vi "PH_ImageOperator.FF MaxEnergy.vi"(0 "i ref in":refnum<vi>, 1 "Image":T1, 2 "Fill Factor":dbl, 5 "error in (no error)":errorcluster) -> (14 "i ref out":refnum<vi>, 16 "Max. allowed energy (J)":dbl, 17 "Error calculating the Energy?":bool, 19 "error out":errorcluster)   [LabVIEW 2014, in "PH_ImageOperator.lvlib"]
doc: "This VI calculates the maximum allowed energy based on a beam profile, the fill factor and a maximum damage threshold fluence.\nThe image to be fed in must be the binary image generated by the \"Convex Hull\" VI."
uses:
  PH_ImageOperator.lvlib
  <vilib>/vision/Image Controls.llb/IMAQ Image.ctl
  <vilib>/vision/NI_Vision_Development_Module.lvlib
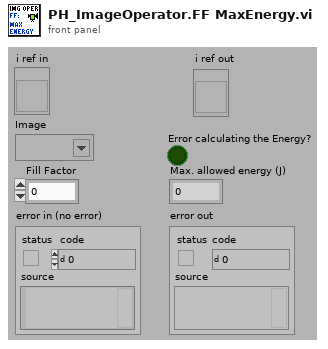
[diagram p1: front panel]
types:
  T1 = typedef "IMAQ Image.ctl" = refnum<image>
  T2 = typedef "PH_ImageOperator.lvlib/PH_ImageOperator.i attribute.ctl" = cluster{"GUI Refs":cluster{"Delete":refnum<vi>, "Calibration status":refnum<vi>, "BI subtracted":refnum<vi>, "calc Energy":refnum<vi>, "Energy: expected value":refnum<vi>, "Energy: Tolerance":refnum<vi>, "Energy calculated":refnum<vi>, "Energy":refnum<vi>, "calc Beam Anal":refnum<vi>, "Maj Diam 1/esquare":refnum<vi>, "Min Diam 1/esquare":refnum<vi>, "Azi Angle":refnum<vi>, "Min/Maj Diam esquare":refnum<vi>, "Beam analysed":refnum<vi>, "CoG - x":refnum<vi>, "CoG - y":refnum<vi>, "BA: Method":refnum<vi>, "BA: Steps":refnum<vi>, "BA: Factor":refnum<vi>, "calc Traces":refnum<vi>, "Traces: Fit Gauss":refnum<vi>, "Traces calculated":refnum<vi>, "Maj FWHM":refnum<vi>, "Min FWHM":refnum<vi>, "Major Trace":refnum<vi>, "Minor Trace":refnum<vi>, "Maj Fit Order":refnum<vi>, "Min Fit Order":refnum<vi>, "Position calculated":refnum<vi>, "Position":refnum<vi>, "Type":refnum<vi>, "Center":refnum<vi>, "exp - X":refnum<vi>, "exp - Y":refnum<vi>, "Tolerance":refnum<vi>, "f":refnum<vi>, "M":refnum<vi>, "D":refnum<vi>, "q":refnum<vi>, "Dummy Method":refnum<vi>, "Dummy Type":refnum<vi>, "Global On":refnum<vi>, "Traces: No offset":refnum<vi>, "Maj 99%":refnum<vi>, "Min 99%":refnum<vi>, "GUI FF Image":refnum<vi>, "calc Fill Factor":refnum<vi>, "FF calculated":refnum<vi>, "Fill Factor: Filter?":refnum<vi>, "FF: Damage Threshold":refnum<vi>, "FF: Threshold":refnum<vi>, "FF: max allow. Energy":refnum<vi>, "FF: Fillfactor":refnum<vi>, "Calibration data":refnum<vi>}, "List of GUIs":string[], "Calibration":cluster{"Status":T3, "Calibration data":T4, "Calibration Data File":path}, "Final Image":cluster{"BI Subtraction Failure":bool}, "Energy":cluster{"on":bool, "expected value [mJ]":dbl, "Tolerance [%]":dbl, "State":T3, "Energy [mJ]":dbl, "Unit":string, "calculated @":timestamp}, "Beam Analysis":cluster{"on":bool, "Data":T5, "Method":bool, "Steps":i32, "Factor":i32, "ROI":cluster{"Left":i32, "Top":i32, "Right":i32, "Bottom":i32}, "analysed @":timestamp}, "Trace Analysis":cluster{"on":bool, "Fit on":bool, "Maj FWHM":dbl, "Min FWHM":dbl, "Maj Fit Order":i32, "Min Fit Order":i32, "No Offset":bool, "Maj 99%":dbl, "Min 99%":dbl, "Traces":cluster{"XScaleName":string, "Y Scale Minimum":sgl, "Y Scale Maximum":sgl, "X Scale Minimum":sgl, "X Scale Maximum":sgl, "Traces":cluster{"Index":sgl[], "Trace":dbl[]}[]}[], "analysed @":timestamp}, "Position Analysis":cluster{"on":bool, "exp - X":i32, "exp - Y":i32, "focal length [mm]":dbl, "Magnification":dbl, "Delta":dbl, "Theta":dbl, "Tolerance":dbl, "Type":bool, "analysed @":timestamp}, "Fill Factor":cluster{"on":bool, "Filter on?":bool, "Threshold":dbl, "Damage Threshold [J/cm²]":dbl, "Fillfactor":dbl, "Max. allowed Energy [J]":dbl, "calculated @":timestamp}, "Statistician Service ID":i32, "Images":cluster{"Background":T1, "OP":T1, "GUI":T1, "BA: ROI":T1, "Trace: Turn":T1, "FF: Main":T1, "FF: Help":T1, "PSDB: BG":T1, "PSDB: OP":T1, "PSDB: FF":T1}}
  T3 = typedef "PH_StatusHandler.lvlib/PH_StatusHandler.Status.ctl" = i16
  T4 = typedef "PH_ImageCalibrator.lvlib/PH_ImageCalibrator.Calibration Data.ctl" = cluster{"Date":string, "Time":string, "Cam Settings":cluster{"Cam ID":string, "Gain":dbl, "Brightness":dbl, "Shutter":dbl, "Cam Error":bool, "Mode":i32}, "Background Image":cluster{"Image":dbl[][], "Image Error":bool}, "Linear Calibration":cluster{"Calibration Factor":dbl, "not mm or mrad":bool}, "Energy Calibration":cluster{"Calibration Factor":dbl, "no mJ":bool}}
  T5 = typedef "PH_ImageOperator.lvlib/PH_ImageOperator.Beam Analysis Data.ctl" = cluster{"CoG-x":sgl, "CoG-y":sgl, "Maj Dim":dbl, "Min Dim":dbl, "Ellipticity":dbl, "Azimuth Angle [rad]":dbl, "Azi Angle rel to Maj?":bool}
  T6 = cluster{"histogram":u32[], "Minimal Value":sgl, "Maximal Value":sgl, "Starting Value":sgl, "Interval Width":sgl, "Mean Value":sgl, "Standard  Variation":sgl, "Area (pixels)":i32}
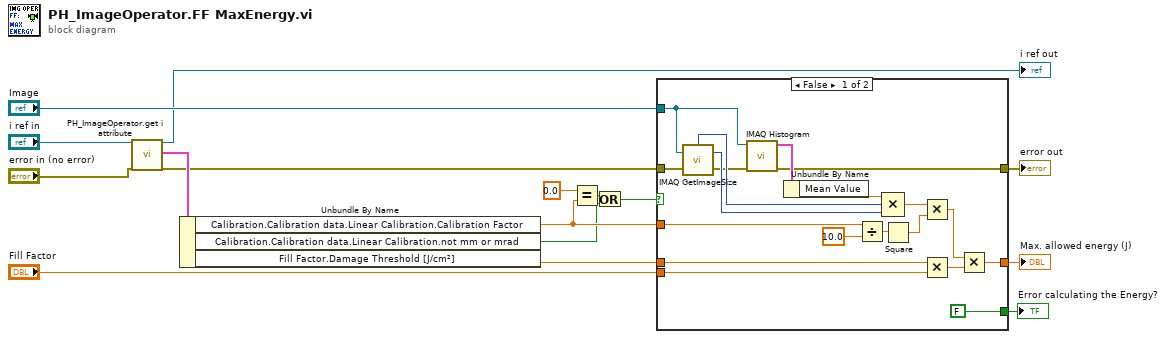
[diagram p0: block diagram]
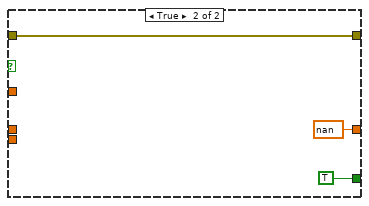
[diagram p2: hidden frame]
diagram:
  n1 = call "PH_ImageOperator.get i attribute.vi"("i ref in"="i ref in", "error in (no error)"="error in (no error)") -> ("i ref out"=→"i ref out":refnum<vi>, "i attribute"=w14:T2, "error out"=w12:errorcluster)  [unwired: 15 in]
  n2 = Unbundle By Name(w14) -> ("Calibration.Calibration data.Linear Calibration.Calibration Factor"=w6:dbl, "Calibration.Calibration data.Linear Calibration.not mm or mrad"=w3:bool, "Fill Factor.Damage Threshold [J/cm²]"=w10:dbl)
  n3 = Equal?(x=0.0, y=w6) -> (x = y?=w4:bool)
  n4 = Or(x=w4, y=w3) -> (x .or. y?=w2:bool)
  n5 = case shown="False" w2 {
    tunnel: [w35 nan ("x")] -> w16
    tunnel: [w25 w38] -> w15
    tunnel: w6 -> [w24 _]
    tunnel: w12 -> [w21 w38]
    tunnel: w10 -> [w20 _]
    tunnel: "Fill Factor" -> [w19 _]
    tunnel: "Image" -> [w18 _]
    tunnel: [FALSE TRUE] -> w1
    frame False {
      n6 = call "IMAQ GetImageSize"("Image"=w18, "error in (no error)"=w21) -> ("Y Resolution"=w30:i32, "X Resolution"=w29:i32, "error out"=w28:errorcluster)  [unwired: 2 in]
      n7 = call "IMAQ Histogram"("error in (no error)"=w28, "Image"=w18) -> ("error out"=w25:errorcluster, "Histogram Report"=w26:T6)  [unwired: 8 in]
      n8 = Unbundle By Name(w26) -> ("Mean Value"=w27:sgl)
      n9 = Divide(x=w24, y=10.0) -> (x/y=w22:dbl)
      n10 = Compound Arithmetic op=MULTIPLY(w27, w29, w30) -> (w31:sgl)
      n11 = Square(x=w22) -> (x^2=w32:dbl)
      n12 = Multiply(x=w31, y=w32) -> (x*y=w34:dbl)
      n13 = Multiply(x=w20, y=w19) -> (x*y=w33:dbl)
      n14 = Multiply(x=w34, y=w33) -> (x*y=w35:dbl)
    }
    frame True {
    }
  }
  "Max. allowed energy (J)" <- w16
  "error out" <- w15
  "Error calculating the Energy?" <- w1
